vi "printStatus.vi"(8 "error in (no error)":errorcluster, 11 "Tv in":refnum<class "Tv.lvclass">) -> (0 "error out":errorcluster, 3 "Tv out":refnum<class "Tv.lvclass">)   [LabVIEW 2017, in "Tv.lvclass"]
uses:
  Tv.lvclass
  ConsoleOut/Print Options.ctl
  Tv.lvclass/Tv.ctl
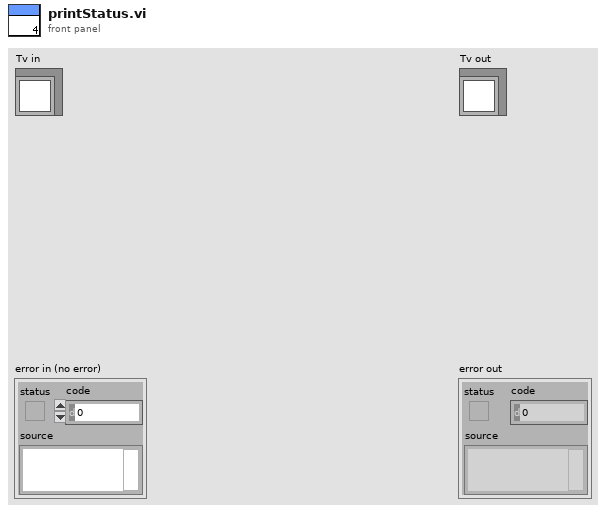
[diagram p1: front panel]
types:
  T1 = typedef "Print Options.ctl" = enum16{"Create", "Get Reference", "Print", "Print Header", "Close"}
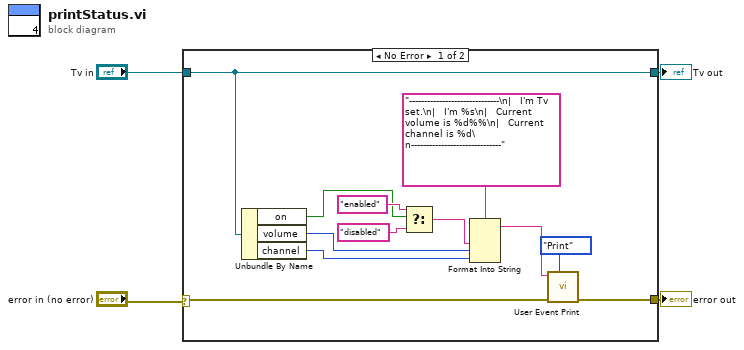
[diagram p0: block diagram]
diagram:
  n1 = case shown="No Error" "error in (no error)" {
    selector: "error in (no error)" -> [w8 w17]
    tunnel: "Tv in" -> [w9 w18]
    tunnel: [w9 w18] -> w3
    tunnel: [w7 w17] -> w1
    frame No Error {
      n2 = Unbundle By Name(w9) -> ("on"=w13:bool, "volume"=w11:i32, "channel"=w10:i32)
      n3 = Select(t="enabled", s=w13, f="disabled") -> (s? t:f=w12:string)
      n4 = Format Into String(format string="------------------------------\n|   I'm Tv set.\n|   I'm %s\n|   Current volume is %d%%\n|   Current channel is %d\n------------------------------", w12, w11, w10) -> (resulting string=w6:string)  [unwired: 2 in, 1 out]
      n5 = call "User Event Print.vi"("Options"=Print_Options."Print", "error in (no error)"=w8, "String to Print"=w6) -> ("error out"=w7:errorcluster)  [unwired: 7 in, 1 out]
    }
    frame Error {
    }
  }
  "error out" <- w1
  "Tv out" <- w3
